vi "channel operation tests.vi"() -> ()   [LabVIEW 2013, in "EthernetIP tests.lvlib"]
uses:
  EthernetIP tests.lvlib
  configuration/EIP Tags Configuration.lvclass
panel:
  out "no error":errorcluster
  out "channels match":bool
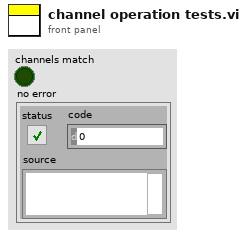
[diagram p1: front panel]
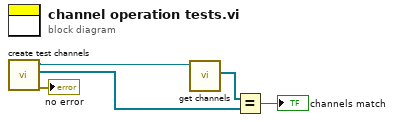
[diagram p0: block diagram]
diagram:
  n1 = call "create test channels.vi"() -> ("error out"=→"no error":errorcluster, "Array"=w2:refnum<class "EIP Tags Channel.lvclass">[], "EthernetIP configuration out"=w3:refnum<class "EIP Tags Configuration.lvclass">)  [unwired: 7 in, 2 out]
  n2 = call-dynamic "get channels.vi"("EthernetIP configuration in"=w3) -> ("channels"=w5:refnum<class "TBM channel.lvclass">[])  [unwired: 9 in, 1 out]
  n3 = Equal?(x=w5, y=w2) -> (x = y?=→"channels match":bool)
